vi "Waveform Flatten and Write.vi"(8 "error in (no error)":errorcluster, 9 "FIFO Timestamps":T1, 10 "Data in":T2[](array[typedef])) -> (0 "error out":errorcluster, 1 "Total Length":i32, 2 "Data out":T2[](array[typedef]), 3 "CIFChannels out":refnum<class "CIFChannels.lvclass">)   [LabVIEW 2021]
uses:
  typedef/Datatype Waveform.ctl
  typedef/TimeStamps.ctl
  CIFChannels/CIFChannels.lvclass
  CIFChannels/CIFChannels.lvclass/CIFChannels.ctl
  be24e584-1bb9-4ddb-b1ad-5fa4498d0a1e.vi
  be24e584-1bb9-4ddb-b1ad-5fa4498d0a1e.vi/c28b0ead-42ad-4072-80a2-aca7f2bd7ce3.vi
  Utilities/Flatten Header.vi
  CIFChannels/Utilities/Update FIFO Header.vi
  Utilities/Add Error.vi
  <vilib>/CIF Foundation/CIF Utilities/DataTypes/Flatten U64.vi
  <vilib>/CIF Foundation/CIF Utilities/Time/System Time/Get System Time.vi
  <vilib>/CIF Foundation/CIF Utilities/Errors/Append Error Location.vi
  <vilib>/CIF Foundation/CIF Utilities/Time/System Time/LabVIEW Time to TAI Time.vi
  <vilib>/CIF Foundation/CIF Utilities/DataTypes/DataTypes_CIF_U.lvlib
  <vilib>/CIFChannels/CIFChannelCore.lvlib
  CIF_NIChn/NIChn/CIF_NIChn.lvclass
  CIF_NIChn/FIFO_Power/CIF_NIChn_Fifo_Power.lvclass
  D:/dev/Packages/Channel_Manager/src/CIFChannels/CIFChannels.lvclass
  D:/dev/Packages/Channel_Manager/src/CIF_NIChn/NIChn/CIF_NIChn.lvclass
  D:/dev/Packages/Channel_Manager/src/CIF_NIChn/FIFO_Power/CIF_NIChn_Fifo_Power.lvclass
  ChannelCommon.lvlib
panel:
  in  "CIFTag in":refnum<class "CIF_NIChn_Fifo_Power.lvclass">
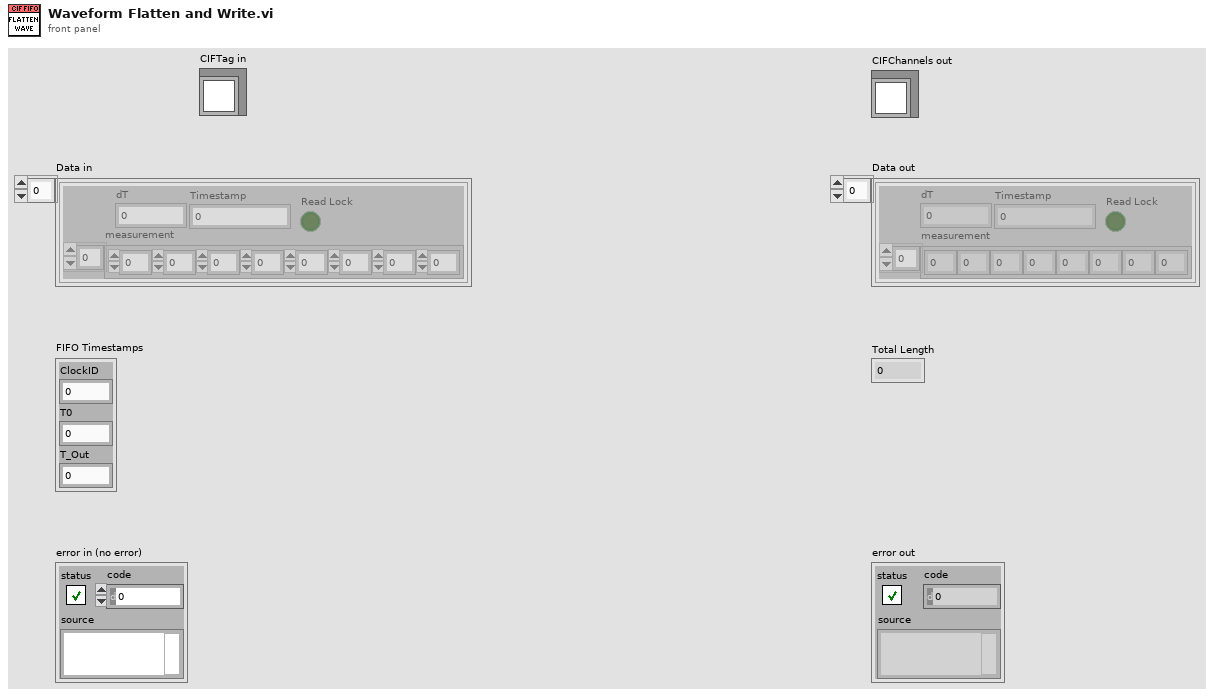
[diagram p1: front panel]
types:
  T1 = typedef "ChannelCommon.lvlib/TimeStamps.ctl" = cluster{"ClockID":u8, "T0":i64, "T_Out":i64}
  T2 = typedef "ChannelCommon.lvlib/Datatype Waveform.ctl" = cluster{"measurement":dbl[], "dT":dbl, "Timestamp":i64, "Read Lock":bool}
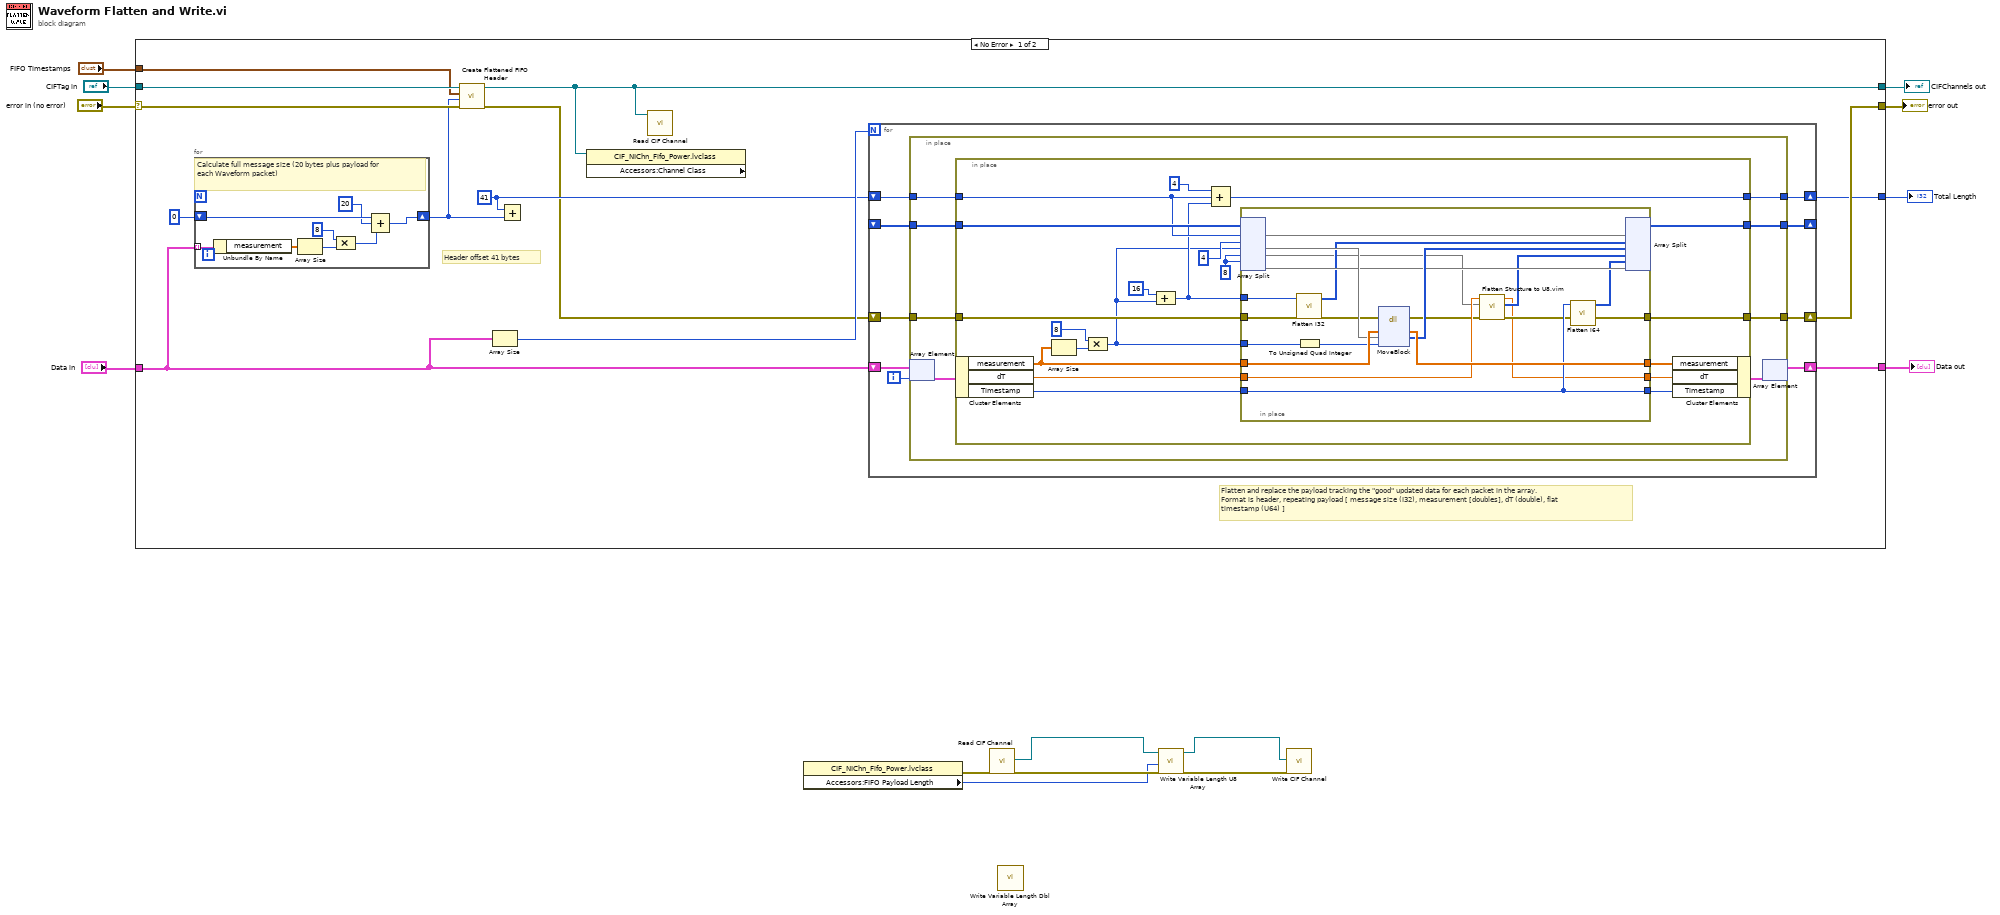
[diagram p0: block diagram]
diagram:
  n1 = case shown="No Error" "error in (no error)" {
    selector: "error in (no error)" -> [w22 w97]
    tunnel: [w29 w97] -> w15
    tunnel: "Data in" -> [w24 w95]
    tunnel: "CIFTag in" -> [w23 w96]
    tunnel: [w17 w96] -> w11
    tunnel: [w28 w95] -> w13
    tunnel: [w26 _] -> w12
    tunnel: "FIFO Timestamps" -> [w18 _]
    frame No Error {
      w27 = 41 ("y")
      # "Flatten and replace the payload tracking the \"good\" updated data for each packet in the array.\nFormat is header, repeating payload [ message size (I32), measurement [doubles], dT (double), flat timestamp (U64) ]"
      # "Header offset 41 bytes"
      n2 = for {
        tunnel: w24 -> [w38] mode=indexing
        shift-right: [w36] -> w21
        shift-left: 0 -> [w35]
        # "Calculate full message size (20 bytes plus payload for each Waveform packet)"
        n3 = Unbundle By Name(w38) -> ("measurement"=w37:dbl[])
        n4 = Array Size(array=w37) -> (size(s)=w33:i32)
        n5 = Compound Arithmetic op=MULTIPLY(8 ("value"), w33) -> (w32:i32)
        n6 = Compound Arithmetic op=ADD(w35, 20 ("value"), w32) -> (w36:i32)
      }
      n7 = call "Create Flattened FIFO Header.vi"("error in (no error)"=w22, "Payload Length"=w21, "FIFO Timestamps"=w18, "CIFChannels in"=w23) -> ("error out"=w19:errorcluster, "CIFChannels out"=w17:refnum<class "CIF_NIChn_Fifo_Power.lvclass">)  [unwired: 5 in, 1 out]
      n8 = Array Size(array=w24) -> (size(s)=w30:i32)
      n9 = Add(x=w27, y=w21) -> ()  [unwired: 1 out]
      n10 = property class="CIF_NIChn_Fifo_Power.lvclass" props=["Accessors:Channel Class"](reference=w17) -> ()  [unwired: 1 in, 3 out]
      n11 = call "Read CIF Channel.vi"("CIFTag in"=w17) -> ()  [unwired: 8 in, 3 out]
      n12 = for {
        N: w30 -> [_]
        shift-right: [w47] -> w29
        shift-left: w19 -> [w46]
        shift-right: [w44] -> _
        shift-left: [w45] -> w20
        shift-right: [w42] -> w26
        shift-left: w27 -> [w43]
        shift-right: [w39] -> w28
        shift-left: w24 -> [w41]
        i -> [w40]
        n13 = in-place {
          in-place-border: [w55] -> w47
          in-place-border: w46 -> [w54]
          in-place-border: w45 -> [w53]
          in-place-border: [w52] -> w44
          in-place-border: w43 -> [w51]
          in-place-border: [w50] -> w42
          n14 = in-place-array #1(w41, w40) -> (w49:T2)
          n15 = in-place {
            in-place-border: [w75] -> w55
            in-place-border: w54 -> [w74]
            in-place-border: w53 -> [w73]
            in-place-border: [w72] -> w52
            in-place-border: w51 -> [w71]
            in-place-border: [w70] -> w50
            w56 = 8
            n16 = in-place-cluster #2(w49) -> ("measurement"=w65:dbl[], "dT"=w64:dbl, "Timestamp"=w63:i64)
            n17 = Array Size(array=w65) -> (size(s)=w58:i32)
            n18 = Compound Arithmetic op=MULTIPLY(8 ("value"), w58) -> (w57:i32)
            n19 = Compound Arithmetic op=ADD(16 ("value"), w57) -> (w67:i32)
            n20 = Compound Arithmetic op=ADD(4, w71, w67) -> (w70:i32)
            n21 = in-place {
              in-place-border: w63 -> [w82]
              in-place-border: w74 -> [w84]
              in-place-border: [w78] -> w75
              in-place-border: w65 -> [w93]
              in-place-border: w64 -> [w81]
              in-place-border: w67 -> [w86]
              in-place-border: [w92] -> w62
              in-place-border: [w76] -> w61
              in-place-border: [w82] -> w60
              in-place-border: w57 -> [w91]
              n22 = in-place-split #3(w73, w71, 4, w57, w56, w56) -> (w94:u8[], w89:u8[], w80:u8[], w87:u8[])  [unwired: 2 out]
              n23 = call <vilib>:"Flatten I32.vi"("I32"=w86) -> ("Flat Data"=w85:u8[])  [unwired: 4 in]
              n24 = To Unsigned Quad Integer(1:w91) -> (0:w90:u64)
              n25 = dll-call lib="LabVIEW" fn="MoveBlock"(error in=w84, "source"=w93, "dest"=w89, "size"=w90) -> (error out=w79:errorcluster, "source"=w92:dbl[], "dest"=w88:u8[])  [unwired: 4 in, 1 out]
              n26 = call "Flatten Structure to U8.vim"("error in"=w79, "Flattened Data in"=w80, "Data to Flatten in"=w81) -> ("error out"=w78:errorcluster, "Flattened Data out"=w77:u8[], "Data to Flatten out"=w76:dbl)  [unwired: 6 in]
              n27 = call <vilib>:"Flatten I64.vi"("I64"=w82) -> ("Flat Data"=w83:u8[])  [unwired: 4 in]
              n28 = in-place-split #3(w94, w85, w88, w77, w83, w87) -> (w72:u8[])  [unwired: 5 out]
            }
            n29 = in-place-cluster #2("measurement"=w62, "dT"=w61, "Timestamp"=w60) -> (w48:T2)
          }
          n30 = in-place-array #1(w48) -> (w39:T2[])  [unwired: 1 out]
        }
      }
    }
    frame Error {
    }
  }
  "error out" <- w15
  "Data out" <- w13
  "Total Length" <- w12
  "CIFChannels out" <- w11
  n31 = property class="CIF_NIChn_Fifo_Power.lvclass"() -> (error out=w5:errorcluster, "Accessors:FIFO Payload Length"=w4:u64)  [unwired: 2 in, 1 out]
  n32 = call "Read CIF Channel.vi"("error in (no error)"=w5) -> ("error out"=w9:errorcluster, "CIF Channel"=w7:refnum<k21>)  [unwired: 8 in, 1 out]
  n33 = call "Write Variable Length Dbl Array.vi"() -> ()  [unwired: 8 in, 4 out]
  n34 = call <vilib>:"Write Variable Length U8 Array.vi"("error in"=w9, "numElements"=w4, "CIF Channel in"=w7) -> ("error out"=w8:errorcluster, "CIF Channel out"=w6:refnum<k21>, "U8 Array in"=w3:u8[])  [unwired: 4 in, 2 out]
  n35 = call "Write CIF Channel.vi"("error in (no error)"=w8, "CIF Channel"=w6) -> ("CIFTag in"=w2:refnum<class "CIF_NIChn.lvclass">)  [unwired: 7 in, 2 out]
